vi "Untitled 1 (SubVI).vi"(10 "Cluster":cluster{"row":i32, "col":i32}, 11 "Maze in":refnum<class "Maze.lvclass">) -> (3 "Maze out":refnum<class "Maze.lvclass">)   [LabVIEW 2021, in "Maze.lvclass"]
uses:
  Maze.lvclass
  Maze.lvclass/Maze.ctl
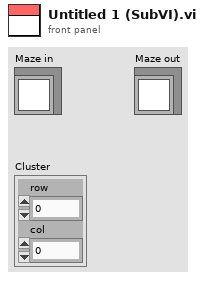
[diagram p1: front panel]
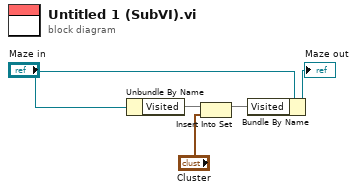
[diagram p0: block diagram]
diagram:
  n1 = Unbundle By Name("Maze in") -> ("Visited"=w4:set{cluster{"row":i32, "col":i32}})
  n2 = Insert Into Set(10:"Cluster", 11:w4) -> (3:w3:set{cluster{"row":i32, "col":i32}})  [unwired: 1 out]
  n3 = Bundle By Name(cluster="Maze in", "Visited"=w3) -> (→"Maze out":refnum<class "Maze.lvclass">)
